vi "DEV test VIs Unwrapped.vi"(8 "Error In":errorcluster) -> (0 "Error Out":errorcluster)   [LabVIEW 2018, in "Receipt Parsing.lvlib"]
uses:
  Receipt Parsing.lvlib
  Action.ctl
panel:
  out "data":string
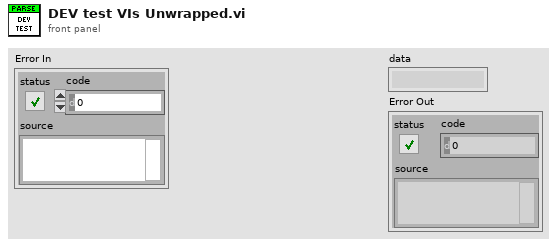
[diagram p1: front panel]
types:
  T1 = typedef "Receipt Parsing.lvlib/Action.ctl" = enum16{"Init", "Read Image Text", "Close"}
  T2 = typedef "IMAQ Image.ctl" = refnum<image>
  T3 = typedef "ROI Descriptor" = cluster{"Global Rectangle":i32[], "Contours":cluster{"ID":enum32{"External", "Internal"}, "Type":u32, "Coordinates":i32[]}[]}
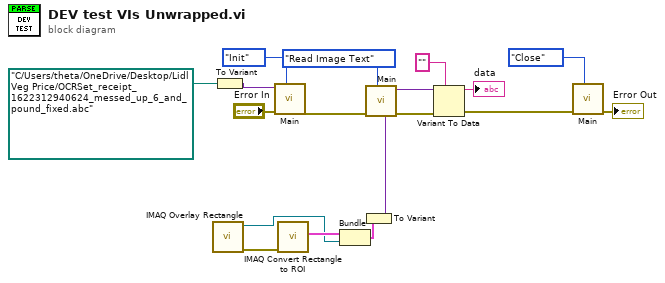
[diagram p0: block diagram]
diagram:
  n1 = call "IMAQ Overlay Rectangle"() -> ("error out"=w12:errorcluster, "Image Out"=w10:T2)  [unwired: 10 in]
  n2 = To Variant(anything=path "C:/Users/theta/OneDrive/Desktop/Lidl Veg Price/OCRSet_receipt_1622312940624_messed_up_6_and_pound_fixed.abc" ("File Path")) -> (Variant=w16:variant)
  n3 = call "Main.vi"("Action"=Action."Init", "Error In"="Error In", "Data In"=w16) -> ("Error Out"=w14:errorcluster)  [unwired: 7 in, 1 out]
  n4 = call "IMAQ Convert Rectangle to ROI"("error in (no error)"=w12) -> ("ROI Descriptor"=w11:T3)  [unwired: 8 in, 1 out]
  n5 = Bundle("ROI Descriptor"=w11, "Image Out"=w10) -> (w9:cluster{"ROI Descriptor":T3, "Image Out":T2})  [unwired: 1 in]
  n6 = To Variant(anything=w9) -> (Variant=w8:variant)
  n7 = call "Main.vi"("Action"=Action."Read Image Text", "Error In"=w14, "Data In"=w8) -> ("Error Out"=w6:errorcluster, "Data Out"=w7:variant)  [unwired: 7 in]
  n8 = Variant To Data(error in=w6, type="", Variant=w7) -> (data=→"data":string, error out=w2:errorcluster)
  n9 = call "Main.vi"("Action"=Action."Close", "Error In"=w2) -> ("Error Out"=→"Error Out":errorcluster)  [unwired: 8 in, 1 out]
